vi "Sub Super Duper_6_14a_JW.vi"(6 "Saved Folder:":path=path "C:/1DATA/2011", 8 "TSP Cluster":T7={"Transport"=FALSE, "Start 2"=0.0, "Stop 3"=-60.0, "Step 2"=-1.0, "Start"=0.0, "Step"=-10.0, "Total Points"=7, "Integration Time"=0} {"Integration Time" scale=0.0..2.0; "Step" format="%.2f"; "Start" format="%.2f"; "Step 2" format="%.2f"; "Stop 3" format="%.2f"; "Start 2" format="%.2f"}, 9 "TRF Cluster":T6={"Step 4"=-38.0, "# of Loops"=1.0, "Transfer 2"=FALSE, "Start 4"=-2.0, "Total Points 2"=2, "Start 3"=40.0, "Stop 2"=-40.0, "Step 3"=-1.0, "Loop Step"=0.0, "Integration Time 3"=0, "Loop Wait"=0.0, "First Step"=0.0} {"Loop Wait" format="%<%H:%M:%S>t"; "Integration Time 3" scale=0.0..2.0; "Step 3" format="%.2f"; "Stop 2" format="%.2f"; "Start 3" format="%.2f"; "Start 4" format="%.2f"; "Step 4" format="%.2f"}, 10 "Sample Properties:":T3 {"Date Created" format="%<%Y/%m/%d>T"}, 11 "Inputs":T8={"VISA resource name"="GPIB0::17::INSTR", "Wait Time (s)"=0.0} {"Wait Time (s)" format="%.1g"}) -> (0 "TSP Path":path, 1 "TRF Path":path, 2 "Char Cluster":T2, 3 "error?":errorcluster, 4 "Wait Countdown":dbl format="%<%H:%M:%S%1u>t", 5 "Graph Cluster":T1)   [LabVIEW 2011]
uses:
  <vilib>/Platform/TimedLoop/XDataNode/timing_clust.ctl
  <vilib>/Platform/TimedLoop/XDataNode/nitl_modes.ctl
  <vilib>/Platform/TimedLoop/XDataNode/wakeup.ctl
  <vilib>/Platform/TimedLoop/XDataNode/XDataNode.xnode
  <vilib>/Platform/TimedLoop/XDataNode/XDNodeRunTimeDep.lvlib
panel:
  in  "Transport Temp":cluster{"trace":dbl[], "trace":dbl[]}(graph)
  in  "Transfer Temp":cluster{dbl[], "trace":dbl[]}[](graph) caption="Transfer"
  out "Boolean":bool
  in  "Stop \nCountdown":bool
  in  "Var2 step settings 2":T4={"compliance (A)"=0.001, "compliance (V)"=100.0} {"compliance (V)" format="%.2f"; "compliance (A)" format="%^.2e"}
  in  "Var1 sweep settings 2":T5={"sweep spacing (linear: 0)"=0, "sweep mode"=FALSE, "compliance (V)"=100.0, "compliance (A)"=0.001} {"compliance (A)" format="%^.2e"; "compliance (V)" format="%.2f"; "sweep spacing (linear: 0)" items=["linear", "log 10", "log 25", "log 50"]}
  in  "Var1 sweep settings":T5={"sweep spacing (linear: 0)"=0, "sweep mode"=FALSE, "compliance (V)"=100.0, "compliance (A)"=0.001} {"compliance (A)" format="%^.2e"; "compliance (V)" format="%.2f"; "sweep spacing (linear: 0)" items=["linear", "log 10", "log 25", "log 50"]}
  in  "Var2 step settings":T4={"compliance (A)"=0.001, "compliance (V)"=100.0} {"compliance (V)" format="%.2f"; "compliance (A)" format="%^.2e"}
  out "graphic display":cluster{"trace":dbl[], "trace":dbl[]}(graph)
  # "Device Characteristics"
  # "Vg Sweep"
  # "Vd Step"
  # "Loops and Integration Time"
  # "Sample Properties:"
  # "%"
  # "nm"
  # "Device Properties:"
  # "um"
  # "um"
  # "Vg Step"
  # "Vd Step"
  # "Integration Time"
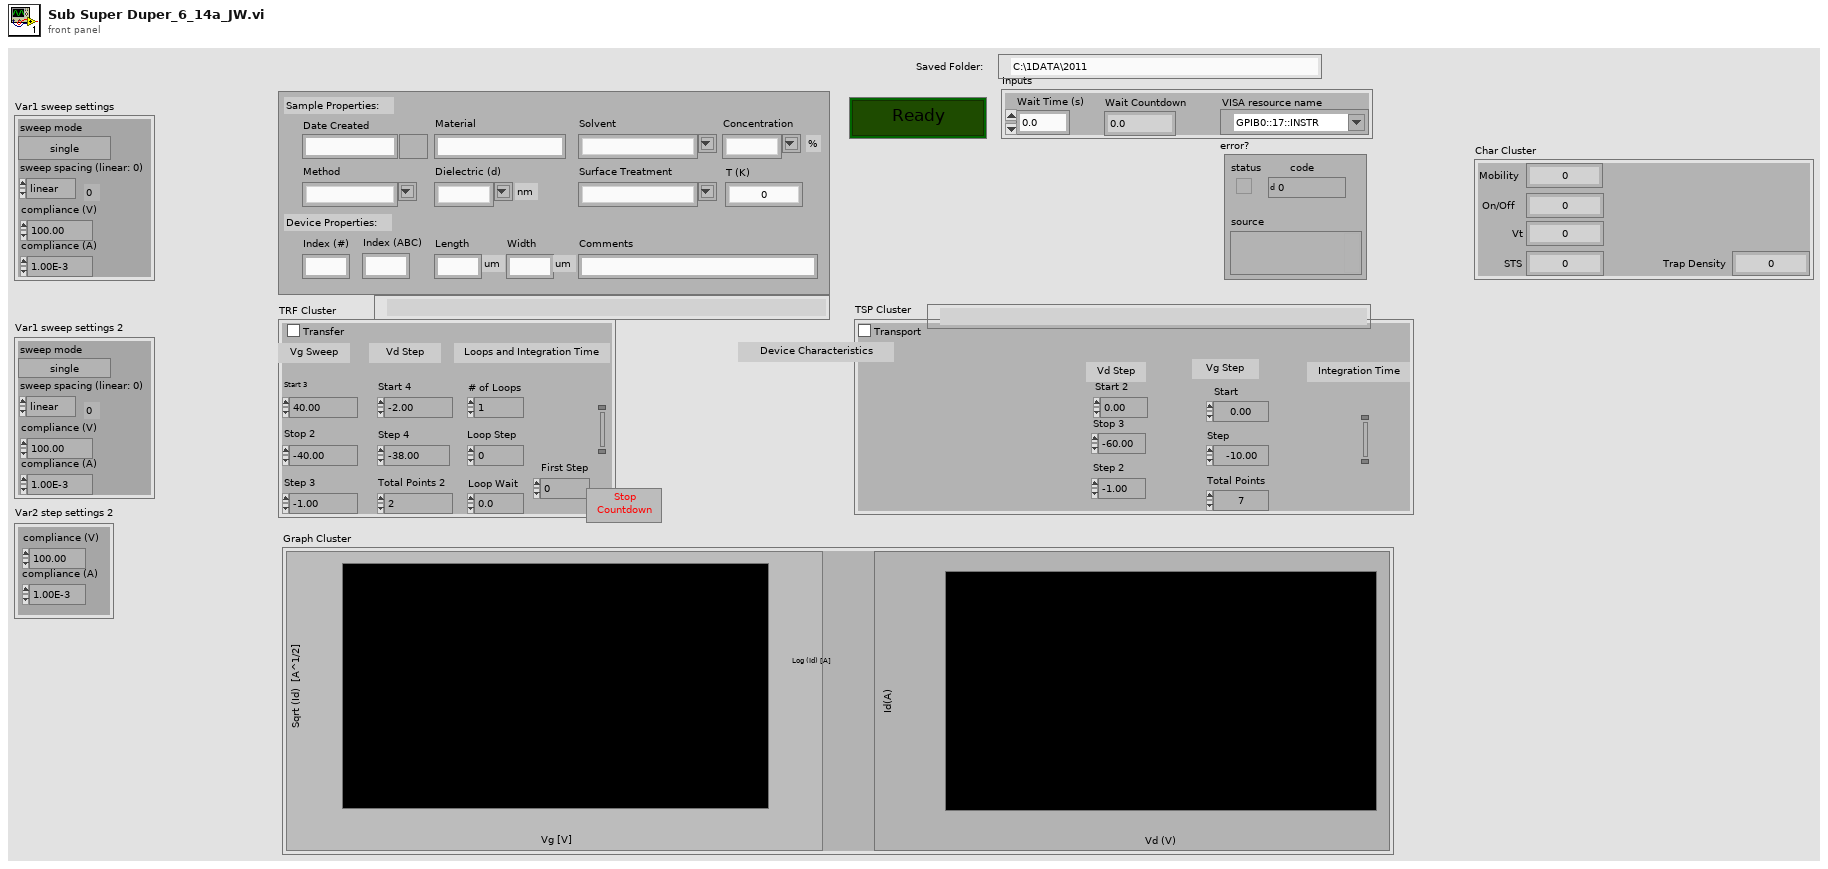
[diagram p1: front panel]
types:
  T1 = cluster{"Transfer":cluster{dbl[], "trace":dbl[]}[], "Transport":cluster{"trace":dbl[], "trace":dbl[]}}
  T2 = cluster{"Mobility":dbl, "On/Off ":dbl, "Vt":dbl, "STS":dbl, "Trap Density":dbl}
  T3 = cluster{"Date Created":timestamp, "Material":string, "Solvent":string, "Concentration":string, "Method":string, "Dielectric (d)":string, "Index (#)":string, "Index (ABC)":string, "Length":string, "Width":string, "Surface Treatment":string, "Comments":string, "T (K)":dbl}
  T4 = cluster{"compliance (A)":dbl, "compliance (V)":dbl}
  T5 = cluster{"sweep spacing (linear: 0)":u16, "sweep mode":bool, "compliance (V)":dbl, "compliance (A)":dbl}
  T6 = cluster{"Step 4":dbl, "# of Loops":dbl, "Transfer 2":bool, "Start 4":dbl, "Total Points 2":u16, "Start 3":dbl, "Stop 2":dbl, "Step 3":dbl, "Loop Step":dbl, "Integration Time 3":u32, "Loop Wait":dbl, "First Step":dbl}
  T7 = cluster{"Transport":bool, "Start 2":dbl, "Stop 3":dbl, "Step 2":dbl, "Start":dbl, "Step":dbl, "Total Points":u16, "Integration Time":u32}
  T8 = cluster{"VISA resource name":refnum<visa-resource-name>, "Wait Time (s)":dbl}
  T9 = typedef "XDNodeRunTimeDep.lvlib/timing_clust.ctl" = cluster{"Expected End [f-1]":u64, "Actual End [f-1]":u64, "Finished Late? [f-1]":bool, "Expected End [i-1]":u64, "Actual End [i-1]":u64, "Finished Late? [i-1]":bool, "Expected Start [i]":u64, "Actual Start [i]":u64, "Expected Start [f]":u64, "Actual Start [f]":u64, "Source Name":string, "Structure Name":string, "Period":i64, "Deadline":i64, "Offset":i64, "Start":i64, "Priority":i32, "Timeout":i32, "Mode":T10, "Wakeup Reason":T11, "Error":errorcluster, "Source Type":string, "Secondary Source Type":string, "Global End Time":u64, "Global Start Time":u64, "Frame Duration":u64, "Iteration Duration":u64, "Assigned CPU":i32, "I/O Scan Engine Mode":u32}
  T10 = typedef "XDNodeRunTimeDep.lvlib/nitl_modes.ctl" = enum32{"No Change", "Process missed periods, maintain original phase", "Discard missed periods, maintain original phase", "Process missed periods, ignore original phase", "Discard missed periods, ignore original phase"}
  T11 = typedef "XDNodeRunTimeDep.lvlib/wakeup.ctl" = enum32{"Normal", "Aborted", "Asynchronous wakeup", "Timing source error", "Timed loop error", "Timeout"}
  T12 = cluster{"Start 3":dbl, "Stop 2":dbl, "Step 3":dbl, "sweep spacing (linear: 0)":u16, "sweep mode":bool, "compliance (V)":dbl, "compliance (A)":dbl}
  T13 = cluster{"compliance (A)":dbl, "compliance (V)":dbl, "Start 4":dbl, "Total Points 2":u16, dbl}
  T14 = cluster{"Step 4":dbl, "# of Loops":dbl, "Transfer 2":bool, "Start 4":dbl, "Total Points 2":u16, "Start 3":dbl, "Stop 2":dbl, "Step 3":dbl, dbl, "Integration Time 3":u32, "Loop Wait":dbl, "First Step":dbl}
  T15 = cluster{"Mobility":dbl, "On/Off Current":dbl, "Vt":dbl, "Trap Density":dbl, "STS":dbl}
  T16 = cluster{"Start 2":dbl, "Stop 3":dbl, "Step 2":dbl, "sweep spacing (linear: 0)":u16, "sweep mode":bool, "compliance (V)":dbl, "compliance (A)":dbl}
  T17 = cluster{"compliance (A)":dbl, "compliance (V)":dbl, "Start":dbl, "Total Points":u16, "Step":dbl}
  T18 = cluster{"Transfer Temp":cluster{dbl[], "trace":dbl[]}[], "Transport Temp":cluster{"trace":dbl[], "trace":dbl[]}}
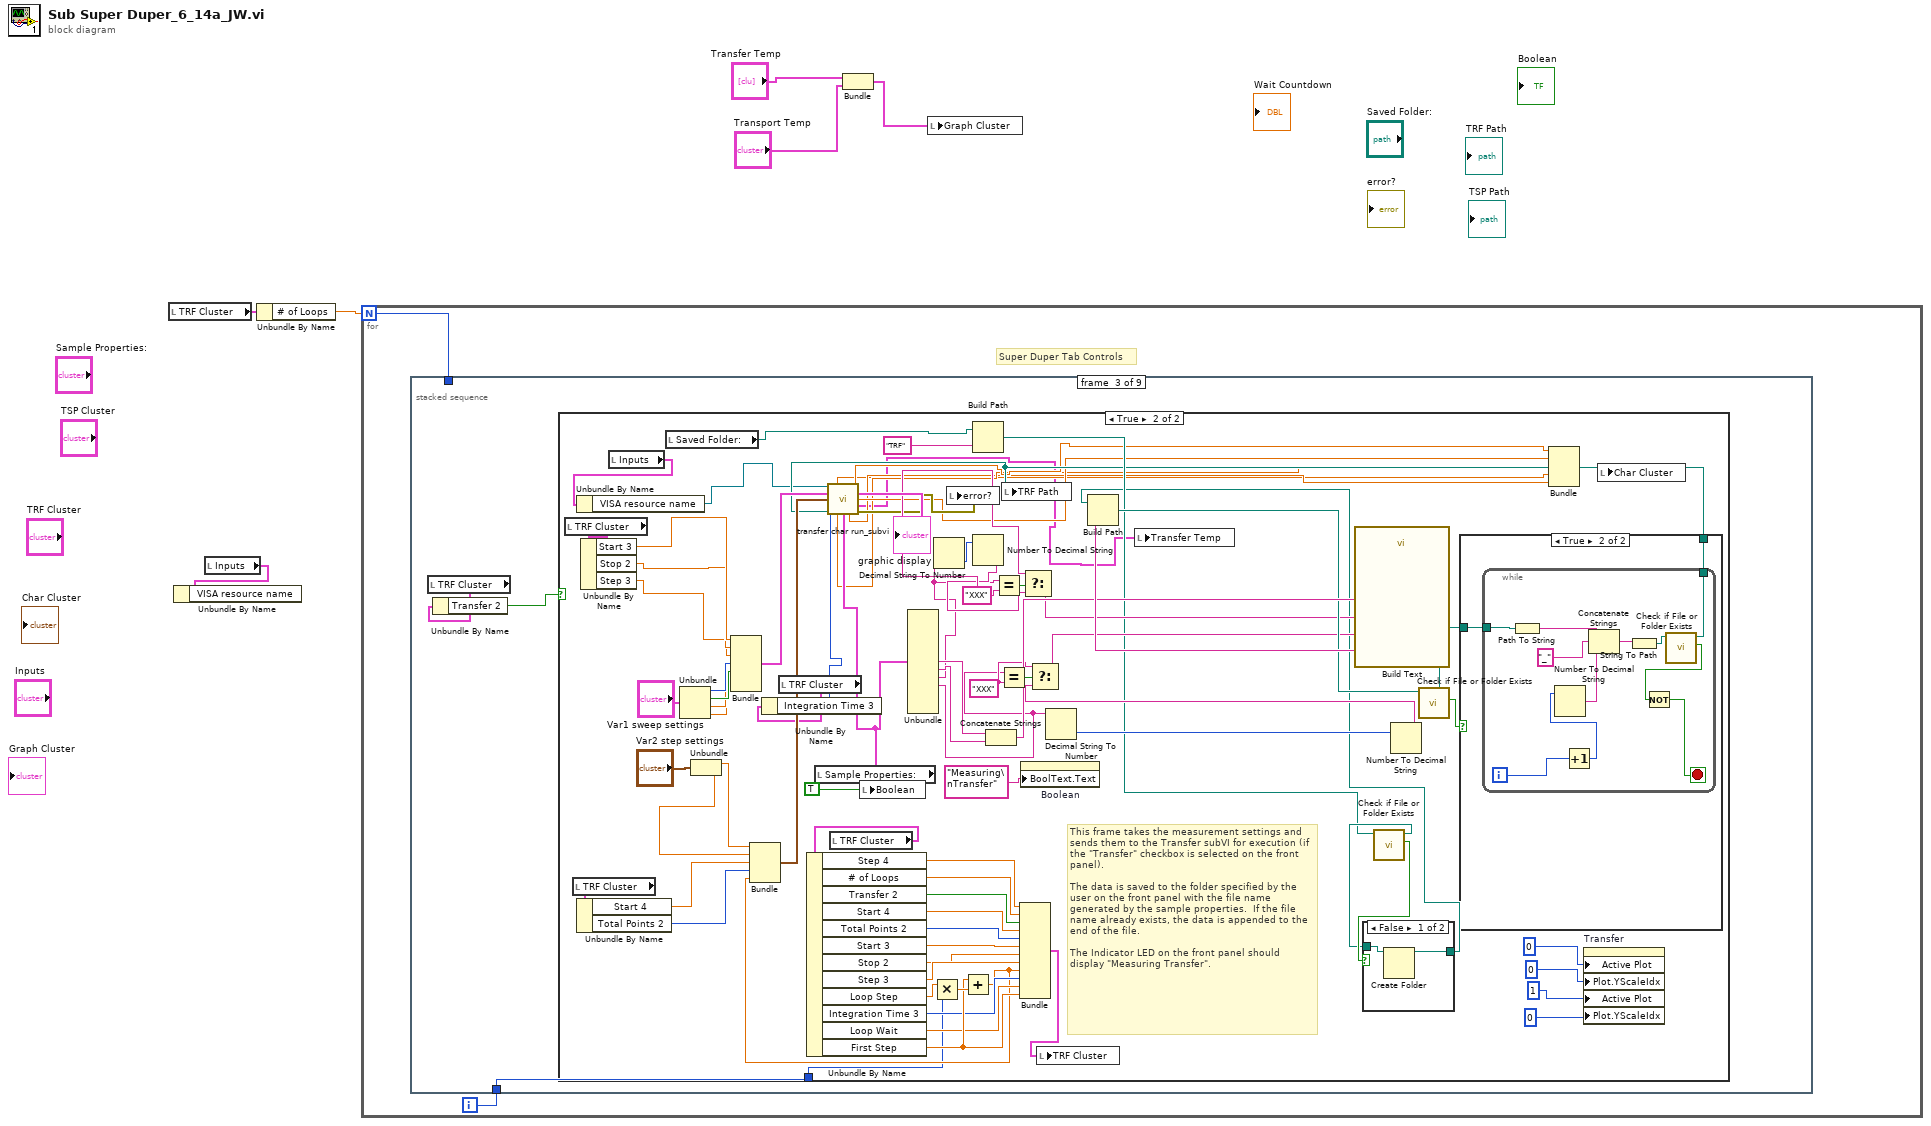
[diagram p0: block diagram]
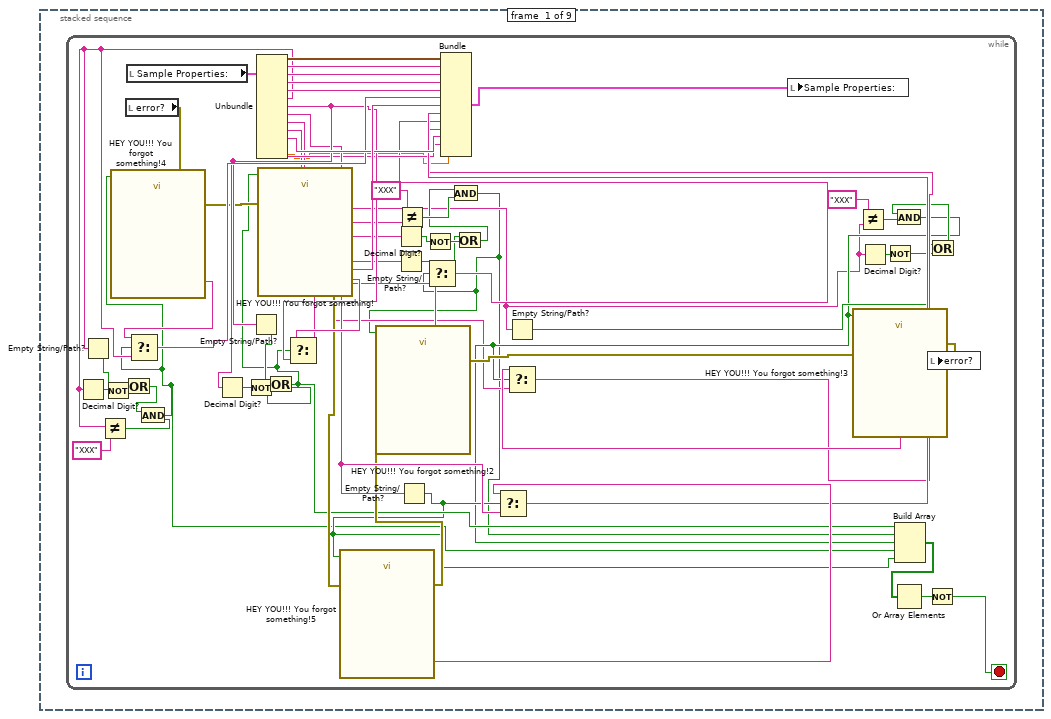
[diagram p2: hidden frame]
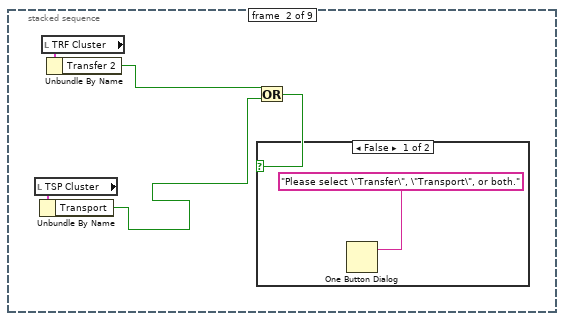
[diagram p3: hidden frame]
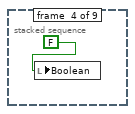
[diagram p8: hidden frame]
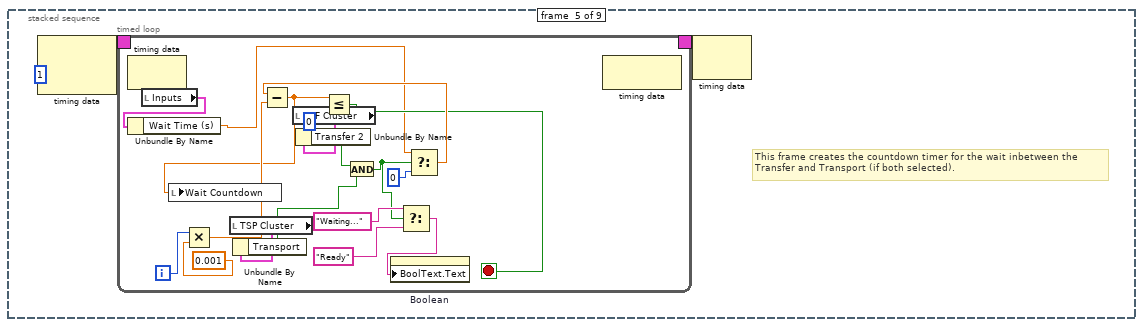
[diagram p9: hidden frame]
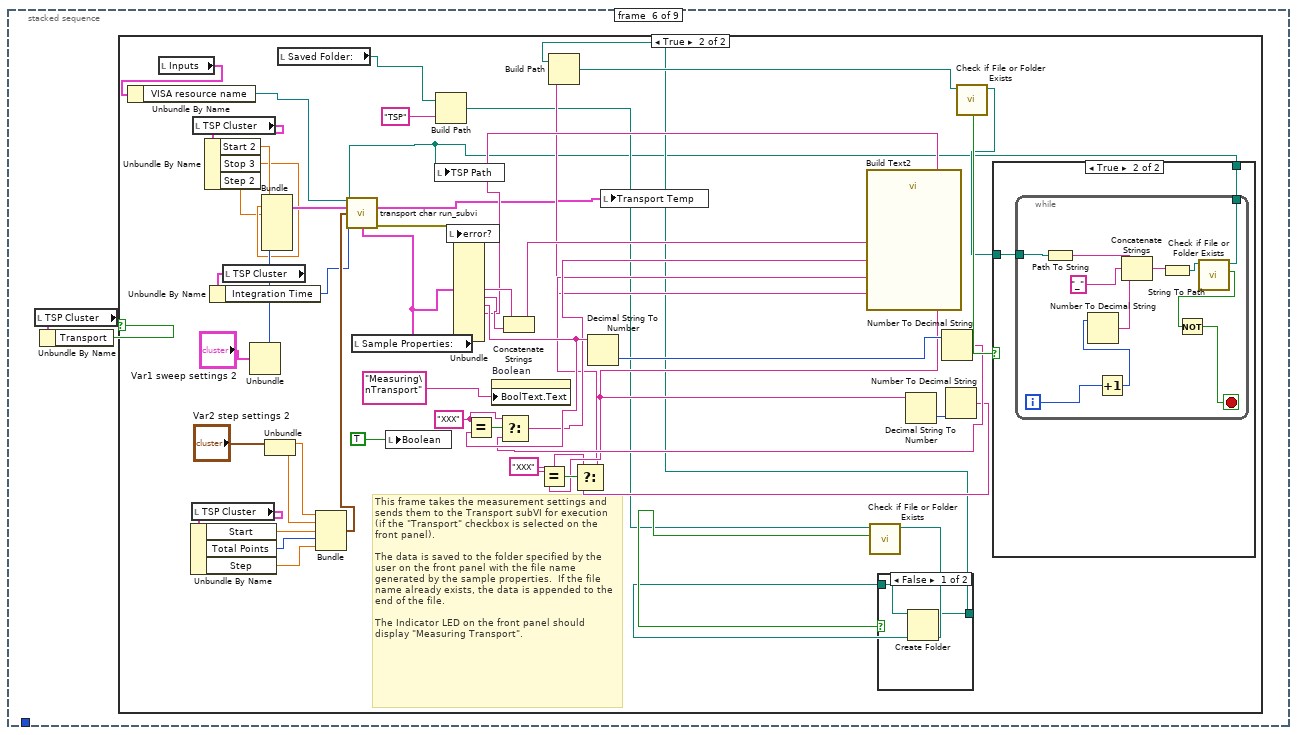
[diagram p10: hidden frame]
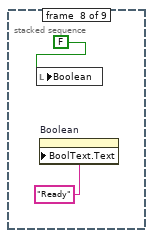
[diagram p15: hidden frame]
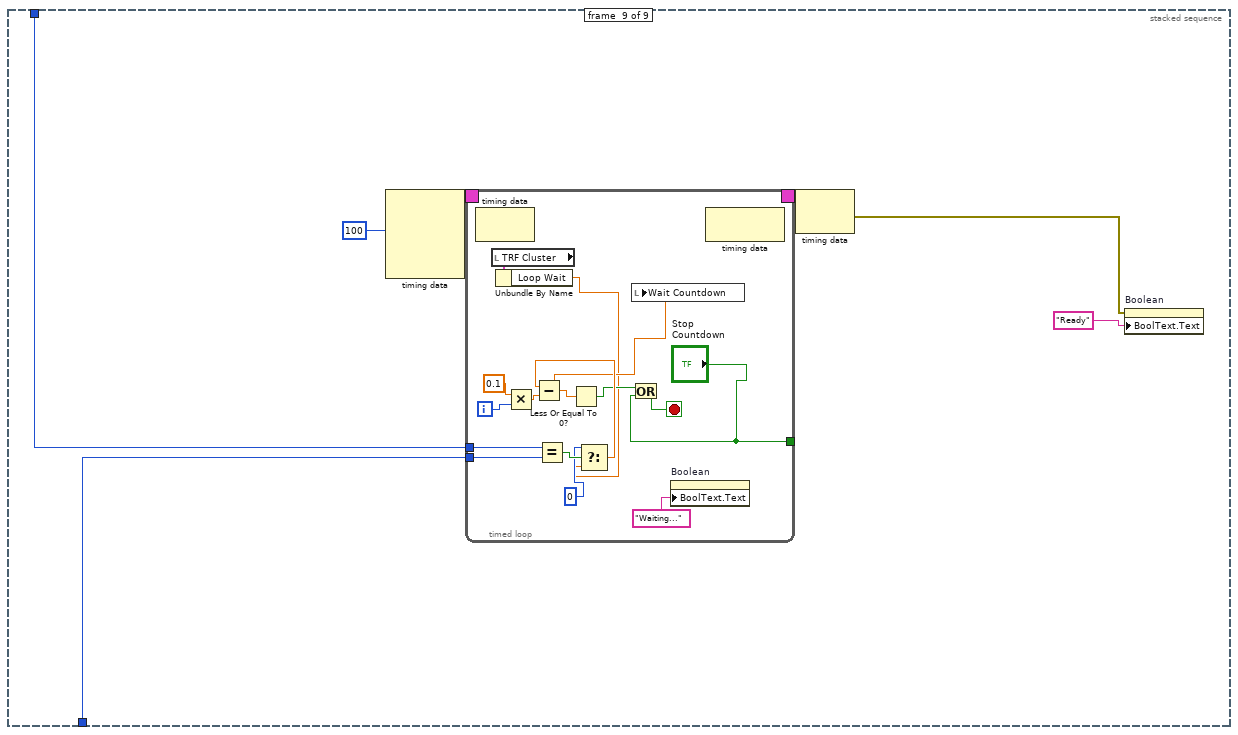
[diagram p16: hidden frame]
diagram:
  n1 = local read "TRF Cluster"() -> (w6:T6)
  n2 = local read "Inputs"() -> (w4:T8)
  n3 = Unbundle By Name(w4) -> ()  [unwired: 1 out]
  n4 = Unbundle By Name(w6) -> ("# of Loops"=w5:dbl)
  n5 = for {
    N: w5 -> [w7]
    i -> [w8]
    # "Super Duper Tab Controls"
    n6 = stacked-sequence {
      tunnel: w8 -> [_ _ w77 _ _ _ _ _ w278]
      tunnel: w7 -> [_ _ _ _ _ _ _ _ w277]
      frame #0 {
        n7 = while {
          stop <- w34 stop-if-true
          n8 = local read "error?"() -> (w40:errorcluster)
          n9 = local read "Sample Properties:"() -> (w63:T3)
          n10 = Unbundle(w63) -> ("Date Created"=w64:timestamp, "Material"=w65:string, "Solvent"=w66:string, "Concentration"=w67:string, "Method"=w68:string, "Dielectric (d)"=w23:string, "Index (#)"=w53:string, "Index (ABC)"=w50:string, "Length"=w18:string, "Width"=w11:string, "Surface Treatment"=w56:string, "Comments"=w48:string, "T (K)"=w9:dbl)
          n11 = Decimal Digit?(1:w23) -> (0:w31:bool)
          n12 = Empty String/Path?(string/path=w23) -> (empty?=w25:bool)
          n13 = Not Equal?(x=w23, y="XXX") -> (x != y?=w22:bool)
          n14 = Not(x=w31) -> (.not. x?=w28:bool)
          n15 = Or(x=w25, y=w28) -> (x .or. y?=w21:bool)
          n16 = And(x=w21, y=w22) -> (x .and. y?=w20:bool)
          n17 = call "HEY YOU!!! You forgot something!4"("Enable"=w20, "error in (no error)"=w40) -> ("Dielectric (d)"=w55:string, "error out"=w39:errorcluster)  [unwired: 15 in, 1 out]
          n18 = Select(t=w55, s=w20, f=w23) -> (s? t:f=w54:string)
          n19 = Decimal Digit?(1:w53) -> (0:w44:bool)
          n20 = Not(x=w44) -> (.not. x?=w43:bool)
          n21 = Empty String/Path?(string/path=w53) -> (empty?=w52:bool)
          n22 = Or(x=w52, y=w43) -> (x .or. y?=w38:bool)
          n23 = call "HEY YOU!!! You forgot something!"("Enable"=w38, "error in (no error)"=w39) -> ("Index (#)"=w62:string, "error out"=w42:errorcluster)  [unwired: 15 in, 1 out]
          n24 = Select(t=w62, s=w38, f=w53) -> (s? t:f=w59:string)
          n25 = Decimal Digit?(1:w18) -> (0:w33:bool)
          n26 = Empty String/Path?(string/path=w18) -> (empty?=w27:bool)
          n27 = Not Equal?(x="XXX", y=w18) -> (x != y?=w17:bool)
          n28 = Empty String/Path?(string/path=w50) -> (empty?=w37:bool)
          n29 = call "HEY YOU!!! You forgot something!5"("Enable"=w37, "error in (no error)"=w42) -> ("Index (ABC)"=w51:string, "error out"=w41:errorcluster)  [unwired: 15 in, 1 out]
          n30 = Not(x=w33) -> (.not. x?=w30:bool)
          n31 = Or(x=w27, y=w30) -> (x .or. y?=w16:bool)
          n32 = And(x=w16, y=w17) -> (x .and. y?=w10:bool)
          n33 = call "HEY YOU!!! You forgot something!2"("Enable"=w10, "error in (no error)"=w41) -> ("Length"=w61:string, "error out"=w58:errorcluster)  [unwired: 15 in, 1 out]
          n34 = Select(t=w61, s=w10, f=w18) -> (s? t:f=w47:string)
          n35 = Select(t=w51, s=w37, f=w50) -> (s? t:f=w49:string)
          n36 = Empty String/Path?(string/path=w11) -> (empty?=w26:bool)
          n37 = Not Equal?(x="XXX", y=w11) -> (x != y?=w15:bool)
          n38 = Decimal Digit?(1:w11) -> (0:w32:bool)
          n39 = Not(x=w32) -> (.not. x?=w29:bool)
          n40 = Or(x=w26, y=w29) -> (x .or. y?=w14:bool)
          n41 = And(x=w14, y=w15) -> (x .and. y?=w13:bool)
          n42 = call "HEY YOU!!! You forgot something!3"("Enable"=w13, "error in (no error)"=w58) -> ("Width"=w60:string, "error out"=w57:errorcluster)  [unwired: 15 in, 1 out]
          n43 = Select(t=w60, s=w13, f=w11) -> (s? t:f=w46:string)
          n44 = Bundle("Date Created"=w64, "Material"=w65, "Solvent"=w66, "Concentration"=w67, "Method"=w68, "Dielectric (d)"=w54, "Index (#)"=w59, "Index (ABC)"=w49, "Length"=w47, "Width"=w46, "Surface Treatment"=w56, "Comments"=w48, "T (K)"=w9) -> (w45:T3)  [unwired: 1 in]
          n45 = local write "Sample Properties:"(w45) -> ()
          n46 = Build Array(w38, w10, w13, w20, w37) -> (w36:bool[])
          n47 = Or Array Elements(Boolean array=w36) -> (logical OR=w35:bool)
          n48 = Not(x=w35) -> (.not. x?=w34:bool)
          n49 = local write "error?"(w57) -> ()
        }
      }
      frame #1 {
        n50 = local read "TSP Cluster"() -> (w70:T7)
        n51 = Unbundle By Name(w70) -> ("Transport"=w69:bool)
        n52 = local read "TRF Cluster"() -> (w72:T6)
        n53 = Unbundle By Name(w72) -> ("Transfer 2"=w71:bool)
        n54 = Or(x=w71, y=w69) -> (x .or. y?=w73:bool)
        n55 = case shown="False" w73 {
          frame False {
            n56 = One Button Dialog(message="Please select \"Transfer\", \"Transport\", or both.") -> ()  [unwired: 1 in, 1 out]
          }
          frame True {
          }
        }
      }
      frame #2 {
        n57 = local read "TRF Cluster"() -> (w75:T6)
        n58 = Unbundle By Name(w75) -> ("Transfer 2"=w76:bool)
        n59 = case shown="True" w76 {
          tunnel: w77 -> [_ w87]
          frame False {
          }
          frame True {
            w130 = "XXX"
            w134 = "XXX"
            # "This frame takes the measurement settings and sends them to the Transfer subVI for execution (if the \"Transfer\" checkbox is selected on the front panel).\n\nThe data is saved to the folder specified by the user on the front panel with the file name generated by the sample properties.  If the file name already exists, the data is appended to the end of the file.\n\nThe Indicator LED on the front panel should display \"Measuring Transfer\"."
            n60 = local read "TRF Cluster"() -> (w109:T6)
            n61 = local read "TRF Cluster"() -> (w113:T6)
            n62 = Unbundle By Name(w113) -> ("Start 4"=w112:dbl, "Total Points 2"=w111:u16)
            n63 = Unbundle By Name(w109) -> ("Start 3"=w108:dbl, "Stop 2"=w107:dbl, "Step 3"=w106:dbl)
            n64 = local read "Inputs"() -> (w80:T8)
            n65 = Unbundle By Name(w80) -> ("VISA resource name"=w79:refnum<visa-resource-name>)
            n66 = local read "Saved Folder:"() -> (w110:path)
            n67 = Unbundle("Var1 sweep settings") -> ("sweep spacing (linear: 0)"=w156:u16, "sweep mode"=w155:bool, "compliance (V)"=w154:dbl, "compliance (A)"=w153:dbl)
            n68 = Unbundle("Var2 step settings") -> ("compliance (A)"=w150:dbl, "compliance (V)"=w149:dbl)
            n69 = Bundle("Start 3"=w108, "Stop 2"=w107, "Step 3"=w106, "sweep spacing (linear: 0)"=w156, "sweep mode"=w155, "compliance (V)"=w154, "compliance (A)"=w153) -> (w152:T12)  [unwired: 1 in]
            n70 = local read "TRF Cluster"() -> (w104:T6)
            n71 = Unbundle By Name(w104) -> ("Integration Time 3"=w105:u32)
            n72 = local read "Sample Properties:"() -> (w116:T3)
            n73 = local read "TRF Cluster"() -> (w90:T6)
            n74 = Unbundle By Name(w90) -> ("Step 4"=w91:dbl, "# of Loops"=w92:dbl, "Transfer 2"=w93:bool, "Start 4"=w94:dbl, "Total Points 2"=w95:u16, "Start 3"=w96:dbl, "Stop 2"=w97:dbl, "Step 3"=w98:dbl, "Loop Step"=w101:dbl, "Integration Time 3"=w99:u32, "Loop Wait"=w100:dbl, "First Step"=w102:dbl)
            n75 = local write "Boolean"(TRUE) -> ()
            n76 = Unbundle(w116) -> ("Index (#)"=w143:string, "Index (ABC)"=w142:string, "Length"=w126:string, "Width"=w129:string)  [unwired: 9 out]
            n77 = Multiply(x=w101, y=w87) -> (x*y=w103:dbl)
            n78 = Decimal String To Number(string=w126) -> (number=w137:i32)  [unwired: 2 in, 1 out]
            n79 = Add(x=w102, y=w103) -> (x+y=w89:dbl)
            n80 = Bundle("compliance (A)"=w150, "compliance (V)"=w149, "Start 4"=w112, "Total Points 2"=w111, w89) -> (w148:T13)  [unwired: 1 in]
            n81 = Build Path(base path=w110, name or relative path="TRF") -> (appended path=w122:path)
            n82 = Number To Decimal String(number=w137) -> (decimal integer string=w133:string)  [unwired: 1 in]
            n83 = Concatenate Strings(w143, w142) -> (w141:string)
            n84 = Equal?(x=w126, y=w134) -> (x = y?=w135:bool)
            n85 = Equal?(x=w129, y=w130) -> (x = y?=w131:bool)
            n86 = Bundle ("Bundle Again")("Step 4"=w91, "# of Loops"=w92, "Transfer 2"=w93, "Start 4"=w94, "Total Points 2"=w95, "Start 3"=w96, "Stop 2"=w97, "Step 3"=w98, w89, "Integration Time 3"=w99, "Loop Wait"=w100, "First Step"=w102) -> (w88:T14)  [unwired: 1 in]
            n87 = property on="Boolean" class="Bool (strict)"("BoolText.Text"="Measuring\nTransfer") -> ()  [unwired: 2 in, 2 out]
            n88 = Select(t=w134, s=w135, f=w133) -> (s? t:f=w132:string)
            n89 = local write "TRF Cluster"(w88) -> ()
            n90 = Decimal String To Number(string=w129) -> (number=w136:i32)  [unwired: 2 in, 1 out]
            n91 = call <vilib>:"Check if File or Folder Exists.vi"("path"=w122) -> ("file or folder exists?"=w124:bool, "dup path"=w123:path)  [unwired: 8 in, 1 out]
            n92 = case shown="False" w124 {
              tunnel: w123 -> [w159 w160]
              tunnel: [w158 w160] -> w121
              frame False {
                n93 = Create Folder(path (use dialog)=w159) -> (created path=w158:path)  [unwired: 2 in, 2 out]
              }
              frame True {
              }
            }
            n94 = Number To Decimal String(number=w136) -> (decimal integer string=w128:string)  [unwired: 1 in]
            n95 = Select(t=w130, s=w131, f=w128) -> (s? t:f=w127:string)
            n96 = call "Build Text"("Index"=w141, "Length"=w132, "Width"=w127) -> ("Result"=w147:string)  [unwired: 11 in, 1 out]
            n97 = Build Path(base path=w121, name or relative path=w147) -> (appended path=w139:path)
            n98 = call <vilib>:"Check if File or Folder Exists.vi"("path"=w139) -> ("file or folder exists?"=w140:bool, "dup path"=w138:path)  [unwired: 8 in, 1 out]
            n99 = case shown="True" w140 {
              tunnel: w138 -> [w161 w163]
              tunnel: [w161 w162] -> w115
              frame False {
              }
              frame True {
                n100 = while {
                  tunnel: w163 -> [w165]
                  tunnel: [w164] -> w162
                  i -> [w167]
                  stop <- w168 stop-if-true
                  n101 = Path To String(path=w165) -> (string=w174:string)
                  n102 = Increment(x=w167) -> (x+1=w166:i32)
                  n103 = Number To Decimal String(number=w166) -> (decimal integer string=w172:string)  [unwired: 1 in]
                  n104 = Concatenate Strings(w174, "_", w172) -> (w171:string)
                  n105 = String To Path(string=w171) -> (path=w170:path)
                  n106 = call <vilib>:"Check if File or Folder Exists.vi"("path"=w170) -> ("file or folder exists?"=w169:bool, "dup path"=w164:path)  [unwired: 8 in, 1 out]
                  n107 = Not(x=w169) -> (.not. x?=w168:bool)
                }
              }
            }
            n108 = call "transfer char run_subvi.vi"("VISA session"=w79, "Var1 sweep settings"=w152, "Var2 step settings"=w148, "integration time"=w105, "Path"=w115, "Sample Properties:"=w116) -> ("Trap Density"=w81:dbl, "Mobility"=w85:dbl, "graphic display"=→"graphic display":cluster{"trace":dbl[], "trace":dbl[]}, "On/Off Current"=w84:dbl, "XY Graph"=w78:cluster{dbl[], "trace":dbl[]}[], "Vt"=w83:dbl, "STS"=w82:dbl, "error?"=w114:errorcluster)  [unwired: 2 in]
            n109 = local write "error?"(w114) -> ()
            n110 = local write "TRF Path"(w115) -> ()
            n111 = local write "Transfer Temp"(w78) -> ()
            n112 = Bundle("Mobility"=w85, "On/Off Current"=w84, "Vt"=w83, "Trap Density"=w81, "STS"=w82) -> (w86:T15)  [unwired: 1 in]
            n113 = property on="Transfer" class="XYGraph (strict)"("Active Plot"=0, "Plot.YScaleIdx"=0, "Active Plot"=1, "Plot.YScaleIdx"=0) -> ()  [unwired: 2 in, 2 out]
            n114 = local write "Char Cluster"(w86) -> ()
          }
        }
      }
      frame #3 {
        n115 = local write "Boolean"(FALSE) -> ()
      }
      frame #4 {
        # "This frame creates the countdown timer for the wait inbetween the\nTransfer and Transport (if both selected)."
        n116 = node-c288(1) -> (w178:T9)  [unwired: 1 in]
        n117 = timed-loop {
          timing: w178 -> [_]
          timing-out: [_] -> w177
          i -> [w188]
          stop <- w189 stop-if-true
          n118 = node-c288() -> ()  [unwired: 1 in, 1 out]
          n119 = local read "Inputs"() -> (w179:T8)
          n120 = Unbundle By Name(w179) -> ("Wait Time (s)"=w180:dbl)
          n121 = Multiply(x=w188, y=0.001) -> (x*y=w186:dbl)
          n122 = local read "TSP Cluster"() -> (w182:T7)
          n123 = Unbundle By Name(w182) -> ("Transport"=w183:bool)
          n124 = local read "TRF Cluster"() -> (w181:T6)
          n125 = Unbundle By Name(w181) -> ("Transfer 2"=w184:bool)
          n126 = And(x=w184, y=w183) -> (x .and. y?=w193:bool)
          n127 = Select(t="Waiting...", s=w193, f="Ready") -> (s? t:f=w195:string)
          n128 = property on="Boolean" class="Bool (strict)"("BoolText.Text"=w195) -> ()  [unwired: 2 in, 2 out]
          n129 = Select(t=w180, s=w193, f=0) -> (s? t:f=w191:dbl)
          n130 = Subtract(x=w191, y=w186) -> (x-y=w185:dbl)
          n131 = local write "Wait Countdown"(w185) -> ()
          n132 = Less Or Equal?(x=w185, y=0) -> (x <= y?=w189:bool)
          n133 = node-c288() -> ()  [unwired: 1 in, 1 out]
        }
        n134 = node-c288(w177) -> ()  [unwired: 1 out]
      }
      frame #5 {
        n135 = local read "TSP Cluster"() -> (w204:T7)
        n136 = Unbundle By Name(w204) -> ("Transport"=w203:bool)
        n137 = case shown="True" w203 {
          frame False {
          }
          frame True {
            w228 = "XXX"
            w232 = "XXX"
            # "This frame takes the measurement settings and sends them to the Transport subVI for execution (if the \"Transport\" checkbox is selected on the front panel).\n\nThe data is saved to the folder specified by the user on the front panel with the file name generated by the sample properties.  If the file name already exists, the data is appended to the end of the file.\n\nThe Indicator LED on the front panel should display \"Measuring Transport\"."
            n138 = local read "Inputs"() -> (w206:T8)
            n139 = Unbundle By Name(w206) -> ("VISA resource name"=w207:refnum<visa-resource-name>)
            n140 = local read "TSP Cluster"() -> (w208:T7)
            n141 = Unbundle By Name(w208) -> ("Start"=w213:dbl, "Total Points"=w212:u16, "Step"=w211:dbl)
            n142 = local read "TSP Cluster"() -> (w217:T7)
            n143 = Unbundle By Name(w217) -> ("Start 2"=w216:dbl, "Stop 3"=w215:dbl, "Step 2"=w214:dbl)
            n144 = local read "TSP Cluster"() -> (w210:T7)
            n145 = Unbundle By Name(w210) -> ("Integration Time"=w209:u32)
            n146 = Unbundle("Var1 sweep settings 2") -> ("sweep spacing (linear: 0)"=w256:u16, "sweep mode"=w255:bool, "compliance (V)"=w254:dbl, "compliance (A)"=w253:dbl)
            n147 = Bundle("Start 2"=w216, "Stop 3"=w215, "Step 2"=w214, "sweep spacing (linear: 0)"=w256, "sweep mode"=w255, "compliance (V)"=w254, "compliance (A)"=w253) -> (w252:T16)  [unwired: 1 in]
            n148 = Unbundle("Var2 step settings 2") -> ("compliance (A)"=w250:dbl, "compliance (V)"=w249:dbl)
            n149 = local read "Saved Folder:"() -> (w218:path)
            n150 = Bundle("compliance (A)"=w250, "compliance (V)"=w249, "Start"=w213, "Total Points"=w212, "Step"=w211) -> (w248:T17)  [unwired: 1 in]
            n151 = local read "Sample Properties:"() -> (w244:T3)
            n152 = local write "Boolean"(TRUE) -> ()
            n153 = Build Path(base path=w218, name or relative path="TSP") -> (appended path=w221:path)
            n154 = Unbundle(w244) -> ("Index (#)"=w243:string, "Index (ABC)"=w242:string, "Length"=w233:string, "Width"=w229:string)  [unwired: 9 out]
            n155 = Equal?(x=w232, y=w233) -> (x = y?=w234:bool)
            n156 = property on="Boolean" class="Bool (strict)"("BoolText.Text"="Measuring\nTransport") -> ()  [unwired: 2 in, 2 out]
            n157 = Concatenate Strings(w243, w242) -> (w241:string)
            n158 = Equal?(x=w228, y=w229) -> (x = y?=w237:bool)
            n159 = Decimal String To Number(string=w233) -> (number=w236:i32)  [unwired: 2 in, 1 out]
            n160 = call <vilib>:"Check if File or Folder Exists.vi"("path"=w221) -> ("file or folder exists?"=w223:bool, "dup path"=w222:path)  [unwired: 8 in, 1 out]
            n161 = case shown="False" w223 {
              tunnel: w222 -> [w259 w260]
              tunnel: [w258 w260] -> w220
              frame False {
                n162 = Create Folder(path (use dialog)=w259) -> (created path=w258:path)  [unwired: 2 in, 2 out]
              }
              frame True {
              }
            }
            n163 = Decimal String To Number(string=w229) -> (number=w235:i32)  [unwired: 2 in, 1 out]
            n164 = Number To Decimal String(number=w236) -> (decimal integer string=w231:string)  [unwired: 1 in]
            n165 = Select(t=w232, s=w234, f=w231) -> (s? t:f=w230:string)
            n166 = Number To Decimal String(number=w235) -> (decimal integer string=w227:string)  [unwired: 1 in]
            n167 = Select(t=w228, s=w237, f=w227) -> (s? t:f=w226:string)
            n168 = call "Build Text2"("Index"=w241, "Length"=w230, "Width"=w226) -> ("Result"=w225:string)  [unwired: 11 in, 1 out]
            n169 = Build Path(base path=w220, name or relative path=w225) -> (appended path=w238:path)
            n170 = call <vilib>:"Check if File or Folder Exists.vi"("path"=w238) -> ("file or folder exists?"=w240:bool, "dup path"=w239:path)  [unwired: 8 in, 1 out]
            n171 = case shown="True" w240 {
              tunnel: w239 -> [w261 w263]
              tunnel: [w261 w262] -> w219
              frame False {
              }
              frame True {
                n172 = while {
                  tunnel: w263 -> [w265]
                  tunnel: [w264] -> w262
                  i -> [w267]
                  stop <- w268 stop-if-true
                  n173 = Path To String(path=w265) -> (string=w274:string)
                  n174 = Increment(x=w267) -> (x+1=w266:i32)
                  n175 = Number To Decimal String(number=w266) -> (decimal integer string=w272:string)  [unwired: 1 in]
                  n176 = Concatenate Strings(w274, "_", w272) -> (w271:string)
                  n177 = String To Path(string=w271) -> (path=w270:path)
                  n178 = call <vilib>:"Check if File or Folder Exists.vi"("path"=w270) -> ("file or folder exists?"=w269:bool, "dup path"=w264:path)  [unwired: 8 in, 1 out]
                  n179 = Not(x=w269) -> (.not. x?=w268:bool)
                }
              }
            }
            n180 = call "transport char run_subvi.vi"("VISA session"=w207, "Var1 sweep settings"=w252, "Var2 step settings"=w248, "integration time"=w209, "Path"=w219, "Sample Properties:"=w244) -> ("graphic display"=w205:cluster{"trace":dbl[], "trace":dbl[]}, "error?"=w247:errorcluster)  [unwired: 8 in]
            n181 = local write "TSP Path"(w219) -> ()
            n182 = local write "error?"(w247) -> ()
            n183 = local write "Transport Temp"(w205) -> ()
          }
        }
      }
      frame #6 {
      }
      frame #7 {
        n184 = local write "Boolean"(FALSE) -> ()
        n185 = property on="Boolean" class="Bool (strict)"("BoolText.Text"="Ready") -> ()  [unwired: 2 in, 2 out]
      }
      frame #8 {
        n186 = node-c288(100) -> (w283:T9)  [unwired: 3 in]
        n187 = timed-loop {
          timing: w283 -> [_]
          timing-out: [_] -> w282
          tunnel: w278 -> [w293]
          tunnel: w277 -> [w292]
          tunnel: ["Stop \nCountdown"] -> _
          i -> [w298]
          stop <- w287 stop-if-true
          n188 = node-c288() -> ()  [unwired: 1 in, 1 out]
          n189 = local read "TRF Cluster"() -> (w285:T6)
          n190 = Unbundle By Name(w285) -> ("Loop Wait"=w284:dbl)
          n191 = Multiply(x=0.1, y=w298) -> (x*y=w296:dbl)
          n192 = Equal?(x=w292, y=w293) -> (x = y?=w294:bool)
          n193 = Select(t=0, s=w294, f=w284) -> (s? t:f=w290:dbl)
          n194 = Subtract(x=w290, y=w296) -> (x-y=w289:dbl)
          n195 = Less Or Equal To 0?(x=w289) -> (x <= 0?=w288:bool)
          n196 = Or(x=w288, y="Stop \nCountdown") -> (x .or. y?=w287:bool)
          n197 = local write "Wait Countdown"(w289) -> ()
          n198 = property on="Boolean" class="Bool (strict)"("BoolText.Text"="Waiting...") -> ()  [unwired: 2 in, 2 out]
          n199 = node-c288() -> ()  [unwired: 1 in, 1 out]
        }
        n200 = node-c288(w282) -> (w279:errorcluster)
        n201 = property on="Boolean" class="Bool (strict)"(error in=w279, "BoolText.Text"="Ready") -> ()  [unwired: 1 in, 2 out]
      }
    }
  }
  n202 = Bundle("Transfer Temp"="Transfer Temp", "Transport Temp"="Transport Temp") -> (w1:T18)  [unwired: 1 in]
  n203 = local write "Graph Cluster"(w1) -> ()
